vi "GenericPowerSupply.vi"() -> ()   [LabVIEW 2014]
uses:
  common/crest/LabVIEW/LV14/libcommon-crest.lvlib
panel:
  out "OFF":bool
  in  "cuname":string="BTF_SIM/QUATB001"
  out "Boolean array":bool[](array[boolean])
  out "size(s)":i32
  out "alrm out":i64 format="%x"
  out "RESETALARMS":bool
  out "update rate (ms)":i64
  out "last data":string
  out "Live":bool
  in  "SetCurrent":dbl step=0.2
  out "ON":bool
  out "Current":dbl(graph)=10.19439697265625
  out "OPEN":bool
  out "NEG":bool
  out "POS":bool
  out "Alarm":bool
  out "Error":bool
  out "Standby":bool
  out "Operational":bool
  in  "stop":bool
  out "current out":dbl
  in  "!CHAOS WAN url":string="192.168.150.91:8081"
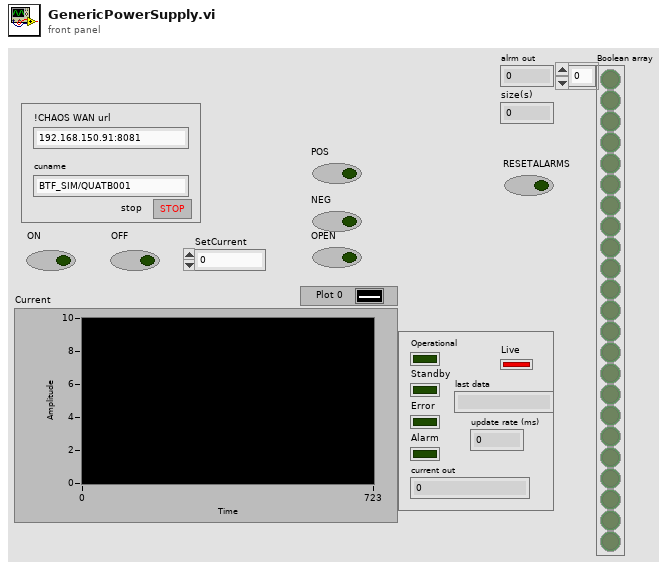
[diagram p1: front panel]
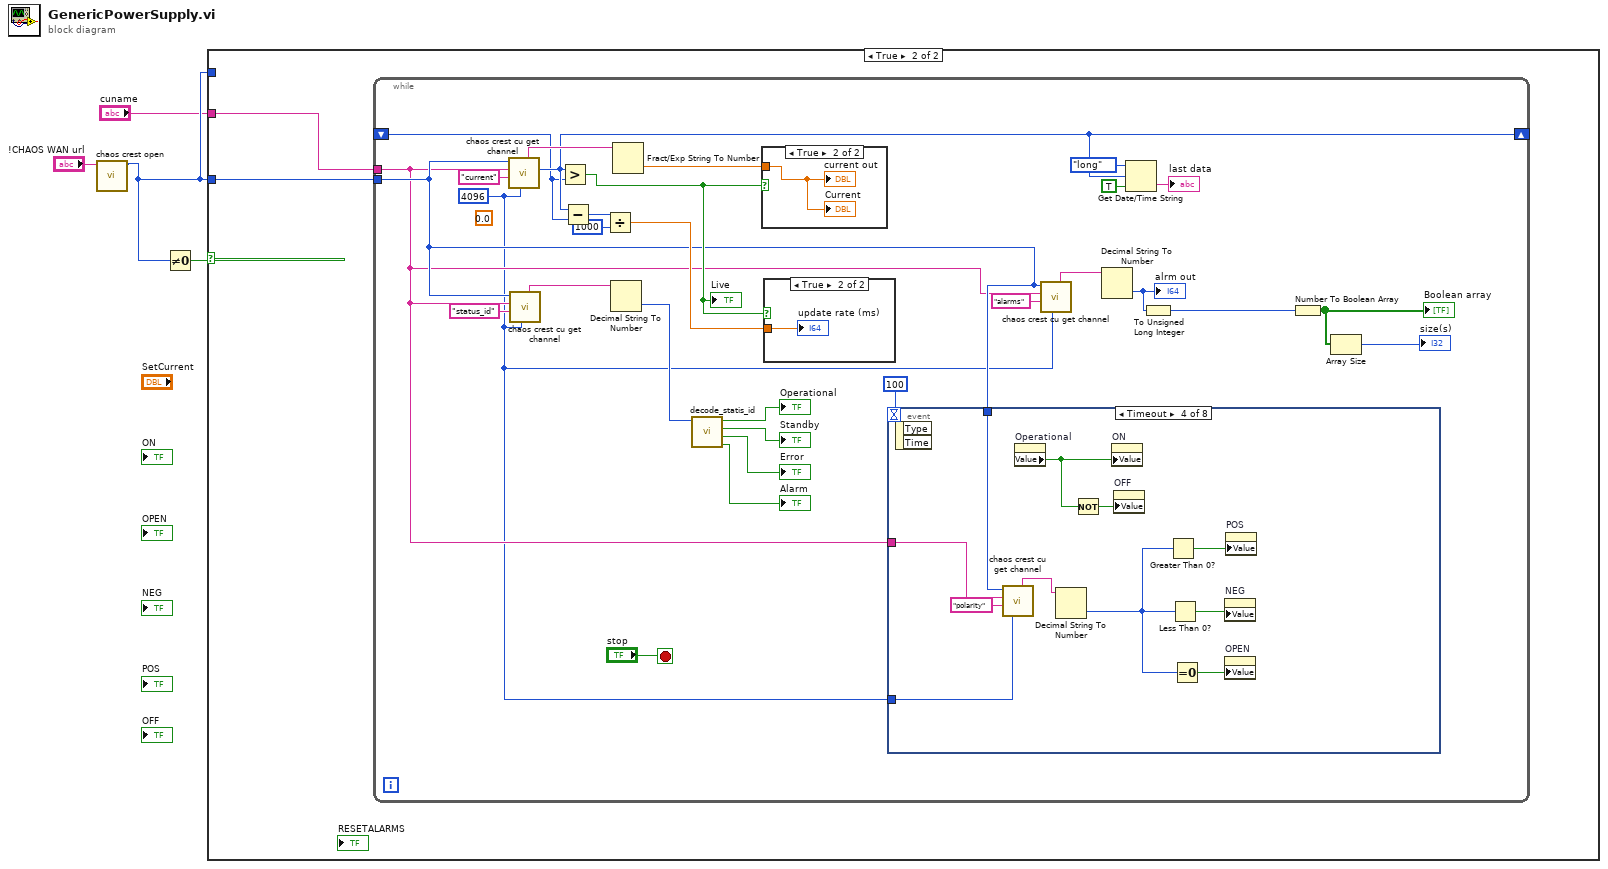
[diagram p0: block diagram]
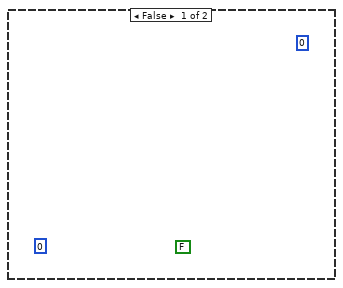
[diagram p2: hidden frame]
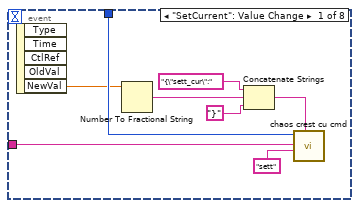
[diagram p4: hidden frame]
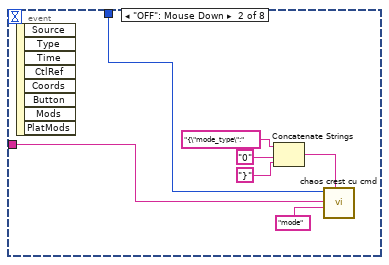
[diagram p5: hidden frame]
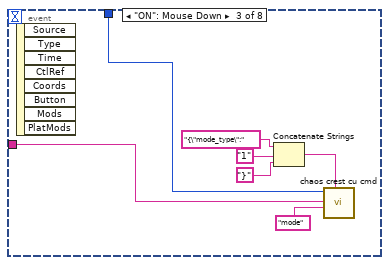
[diagram p6: hidden frame]
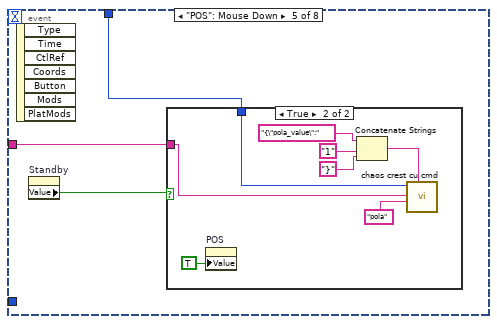
[diagram p7: hidden frame]
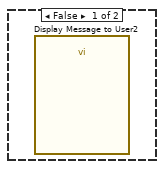
[diagram p8: hidden frame]
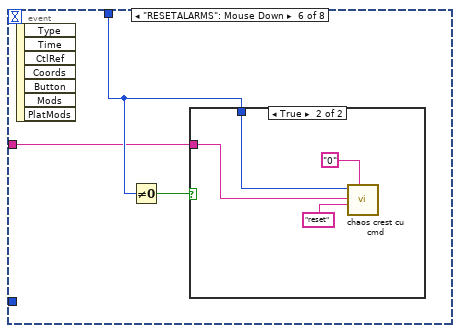
[diagram p9: hidden frame]
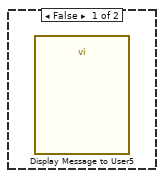
[diagram p10: hidden frame]
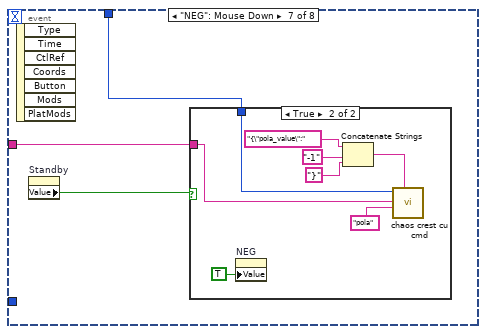
[diagram p11: hidden frame]
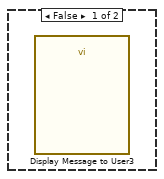
[diagram p12: hidden frame]
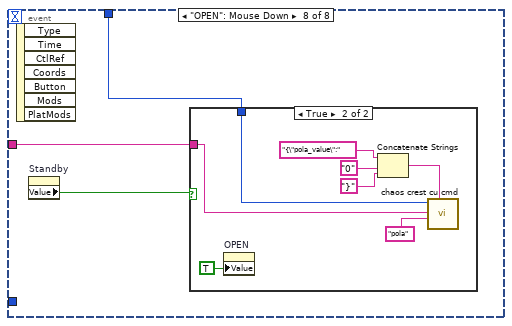
[diagram p13: hidden frame]
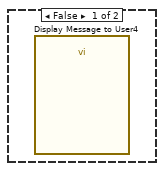
[diagram p14: hidden frame]
diagram:
  n1 = call "chaos crest open.vi"("chaoswanurl"="!CHAOS WAN url") -> ("function return"=w2:u32)  [unwired: 10 in]
  n2 = Not Equal To 0?(x=w2) -> (x != 0?=w4:bool)
  n3 = case shown="True" w4 {
    tunnel: w2 -> [_ w6]
    tunnel: w2 -> [_ _]
    tunnel: "cuname" -> [_ w5]
    frame False {
      (unwired) 0 ("pol out")
      (unwired) 0 ("state out")
      (unwired) FALSE
    }
    frame True {
      n4 = while {
        tunnel: w6 -> [w13]
        shift-right: [w8] -> _
        shift-left: _ -> [w7]
        tunnel: w5 -> [w10]
        stop <- "stop" stop-if-true
        w9 = 4096 ("maxsize")
        (unwired) 0.0 ("current")
        n5 = call "chaos crest cu get channel.vi"("maxsize"=w9, "channame"="current", "cuname"=w10, "h"=w13) -> ("timestamp"=w8:u64, "output out"=w27:string)  [unwired: 5 in, 1 out]
        n6 = call "chaos crest cu get channel.vi"("maxsize"=w9, "channame"="status_id", "cuname"=w10, "h"=w13) -> ("output out"=w16:string)  [unwired: 5 in, 2 out]
        n7 = Greater?(x=w8, y=w7) -> (0:w21:bool)
        "Live" <- w21
        n8 = Subtract(x=w8, y=w7) -> (x-y=w20:u64)
        n9 = Divide(x=w20, y=u32 1000) -> (x/y=w18:dbl)
        n10 = Decimal String To Number(string=w16) -> (number=w15:i32)  [unwired: 2 in, 1 out]
        n11 = Fract/Exp String To Number(string=w27) -> (number=w26:dbl)  [unwired: 3 in, 1 out]
        n12 = call "decode_statis_id.vi"("satatus_id"=w15) -> ("Alarm"=→"Alarm":bool, "Error"=→"Error":bool, "Standby"=→"Standby":bool, "Operational"=→"Operational":bool)  [unwired: 7 in]
        n13 = case shown="True" w21 {
          tunnel: w26 -> [_ w111]
          frame False {
          }
          frame True {
            "Current" <- w111
            "current out" <- w111
          }
        }
        n14 = case shown="True" w21 {
          tunnel: w18 -> [_ w37]
          frame False {
          }
          frame True {
            "update rate (ms)" <- w37
          }
        }
        n15 = event shown="[3] Timeout" {
          selector: _ -> [_ _ _ _ _ _ _ _]
          dyn-events: _ -> [_ _ _ _ _ _ _ _]
          timeout: 100 -> [_ _ _ _ _ _ _ _]
          tunnel: w13 -> [w45 w52 w59 w67 w73 w84 w91 w102]
          tunnel: w10 -> [w43 w51 w58 w64 w71 w82 w89 w100]
          tunnel: w9 -> [_ _ _ w66 _ _ _ _]
          event "SetCurrent": Value Change {
            n16 = event-data() -> ("NewVal"=w41:dbl)  [unwired: 1 in, 4 out]
            n17 = Number To Fractional String(number=w41) -> (F-format string=w40:string)  [unwired: 3 in]
            n18 = Concatenate Strings("{\"sett_cur\":", w40, "}" ("string")) -> (w39:string)
            n19 = call "chaos crest cu cmd.vi"("args"=w39, "cmd"="sett", "cuname"=w43, "h"=w45) -> ()  [unwired: 6 in, 2 out]
          }
          event "OFF": Mouse Down {
            n20 = event-data() -> ()  [unwired: 1 in, 8 out]
            n21 = Concatenate Strings("{\"mode_type\":", "0" ("string"), "}" ("string")) -> (w48:string)
            n22 = call "chaos crest cu cmd.vi"("args"=w48, "cmd"="mode", "cuname"=w51, "h"=w52) -> ()  [unwired: 6 in, 2 out]
          }
          event "ON": Mouse Down {
            n23 = event-data() -> ()  [unwired: 1 in, 8 out]
            n24 = Concatenate Strings("{\"mode_type\":", "1" ("string"), "}" ("string")) -> (w55:string)
            n25 = call "chaos crest cu cmd.vi"("args"=w55, "cmd"="mode", "cuname"=w58, "h"=w59) -> ()  [unwired: 6 in, 2 out]
          }
          event Timeout {
            n26 = event-data() -> ()  [unwired: 1 in, 2 out]
            n27 = call "chaos crest cu get channel.vi"("maxsize"=w66, "channame"="polarity", "cuname"=w64, "h"=w67) -> ("output out"=w63:string)  [unwired: 5 in, 2 out]
            n28 = property on="Operational" class="Bool (strict)"() -> ("Value"=w61:bool)  [unwired: 2 in, 2 out]
            n29 = Decimal String To Number(string=w63) -> (number=w62:i32)  [unwired: 2 in, 1 out]
            n30 = Not(x=w61) -> (.not. x?=w60:bool)
            n31 = property on="ON" class="Bool (strict)"("Value"=w61) -> ()  [unwired: 2 in, 2 out]
            n32 = property on="OFF" class="Bool (strict)"("Value"=w60) -> ()  [unwired: 2 in, 2 out]
            n33 = Greater Than 0?(x=w62) -> (x > 0?=w68:bool)
            n34 = Less Than 0?(x=w62) -> (x < 0?=w69:bool)
            n35 = Equal To 0?(x=w62) -> (x = 0?=w70:bool)
            n36 = property on="NEG" class="Bool (strict)"("Value"=w69) -> ()  [unwired: 2 in, 2 out]
            n37 = property on="OPEN" class="Bool (strict)"("Value"=w70) -> ()  [unwired: 2 in, 2 out]
            n38 = property on="POS" class="Bool (strict)"("Value"=w68) -> ()  [unwired: 2 in, 2 out]
          }
          event "POS": Mouse Down {
            n39 = event-data() -> ()  [unwired: 1 in, 7 out]
            n40 = property on="Standby" class="Bool (strict)"() -> ("Value"=w72:bool)  [unwired: 2 in, 2 out]
            n41 = case shown="True" w72 {
              tunnel: w73 -> [_ w74]
              tunnel: w71 -> [_ w75]
              frame False {
                n42 = call "Display Message to User2"() -> ()  [unwired: 10 in, 2 out]
              }
              frame True {
                n43 = property on="POS" class="Bool (strict)"("Value"=TRUE ("POS")) -> ()  [unwired: 2 in, 2 out]
                n44 = Concatenate Strings("{\"pola_value\":", "1" ("string"), "}" ("string")) -> (w78:string)
                n45 = call "chaos crest cu cmd.vi"("args"=w78, "cmd"="pola", "cuname"=w75, "h"=w74) -> ()  [unwired: 6 in, 2 out]
              }
            }
          }
          event "RESETALARMS": Mouse Down {
            n46 = event-data() -> ()  [unwired: 1 in, 7 out]
            n47 = Not Equal To 0?(x=w84) -> (x != 0?=w83:bool)
            n48 = case shown="True" w83 {
              tunnel: w84 -> [_ w87]
              tunnel: w82 -> [_ w86]
              frame False {
                n49 = call "Display Message to User5"() -> ()  [unwired: 10 in, 2 out]
              }
              frame True {
                n50 = call "chaos crest cu cmd.vi"("args"="0", "cmd"="reset", "cuname"=w86, "h"=w87) -> ()  [unwired: 6 in, 2 out]
              }
            }
          }
          event "NEG": Mouse Down {
            n51 = event-data() -> ()  [unwired: 1 in, 7 out]
            n52 = property on="Standby" class="Bool (strict)"() -> ("Value"=w90:bool)  [unwired: 2 in, 2 out]
            n53 = case shown="True" w90 {
              tunnel: w91 -> [_ w93]
              tunnel: w89 -> [_ w92]
              frame False {
                n54 = call "Display Message to User3"() -> ()  [unwired: 10 in, 2 out]
              }
              frame True {
                n55 = property on="NEG" class="Bool (strict)"("Value"=TRUE ("NEG")) -> ()  [unwired: 2 in, 2 out]
                n56 = Concatenate Strings("{\"pola_value\":", "-1" ("string"), "}" ("string")) -> (w96:string)
                n57 = call "chaos crest cu cmd.vi"("args"=w96, "cmd"="pola", "cuname"=w92, "h"=w93) -> ()  [unwired: 6 in, 2 out]
              }
            }
          }
          event "OPEN": Mouse Down {
            n58 = event-data() -> ()  [unwired: 1 in, 7 out]
            n59 = property on="Standby" class="Bool (strict)"() -> ("Value"=w101:bool)  [unwired: 2 in, 2 out]
            n60 = case shown="True" w101 {
              tunnel: w102 -> [_ w103]
              tunnel: w100 -> [_ w104]
              frame False {
                n61 = call "Display Message to User4"() -> ()  [unwired: 10 in, 2 out]
              }
              frame True {
                n62 = property on="OPEN" class="Bool (strict)"("Value"=TRUE ("OPEN")) -> ()  [unwired: 2 in, 2 out]
                n63 = Concatenate Strings("{\"pola_value\":", "0" ("string"), "}" ("string")) -> (w107:string)
                n64 = call "chaos crest cu cmd.vi"("args"=w107, "cmd"="pola", "cuname"=w104, "h"=w103) -> ()  [unwired: 6 in, 2 out]
              }
            }
          }
        }
        n65 = call "chaos crest cu get channel.vi"("maxsize"=w9, "channame"="alarms", "cuname"=w10, "h"=w13) -> ("output out"=w12:string)  [unwired: 5 in, 2 out]
        n66 = Decimal String To Number(string=w12) -> (number=w11:i32)  [unwired: 2 in, 1 out]
        "alrm out" <- w11
        n67 = Get Date/Time String(date format (0)=enum16{"short", "long", "abbreviated"}."long", seconds (now)=w8, want seconds? (F)=TRUE) -> (time string=→"last data":string)  [unwired: 1 out]
        n68 = To Unsigned Long Integer(number=w11) -> (unsigned 32bit integer=w29:u32)
        n69 = Number To Boolean Array(number=w29) -> (Boolean array=w31:bool[])
        "Boolean array" <- w31
        n70 = Array Size(array=w31) -> (size(s)=→"size(s)":i32)
      }
    }
  }
